vi "TwGetRegUserDataFromH5.vi"(4 "description in":u8[](array[numeric]), 5 "location":string, 6 "buffer in":dbl[](array[numeric]), 7 "filename":string, 8 "bufLength in":i32, 9 "writeIndex":i32, 10 "bufIndex":i32, 11 "error in (no error)":errorcluster) -> (0 "description out":u8[](array[numeric]), 1 "buffer out":dbl[](array[numeric]), 2 "bufLength out":i32, 3 "error out":errorcluster)   [LabVIEW 2009]
uses:
  TwH5Dll.dll
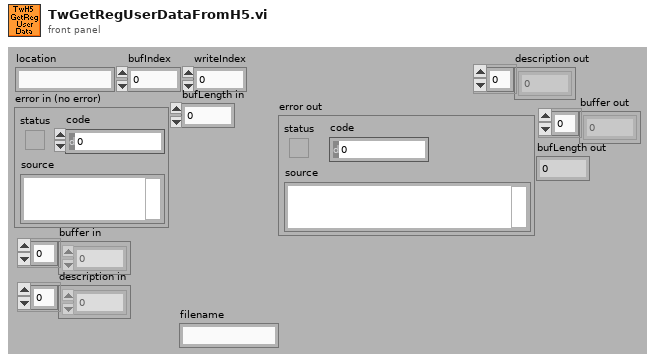
[diagram p1: front panel]
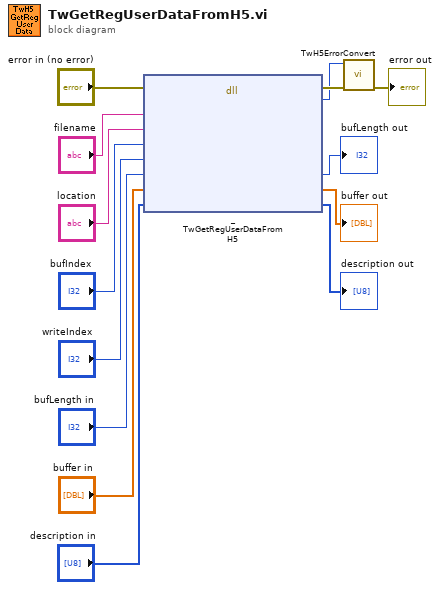
[diagram p0: block diagram]
diagram:
  n1 = dll-call lib="C:/src/85_TofDaq_current/DllWrappers/LabView/TwH5Dll/TwH5Dll.dll" fn="_TwGetRegUserDataFromH5"(error in="error in (no error)", "filename"="filename", "location"="location", "bufIndex"="bufIndex", "writeIndex"="writeIndex", "bufLength"="bufLength in", "buffer"="buffer in", "description"="description in") -> (error out=w13:errorcluster, "TwRetVal"=w12:i32, "bufLength"=→"bufLength out":i32, "buffer"=→"buffer out":dbl[], "description"=→"description out":u8[])  [unwired: 6 in, 1 out]
  n2 = call "TwH5ErrorConvert.vi"("error in (no error)"=w13, "error code"=w12) -> ("error out"=→"error out":errorcluster)  [unwired: 9 out]
